vi "WriteFault.vi"(1 "Fault":T1 {"Severity" max=10}, 2 "FaultDevRef":T3) -> ()   [LabVIEW 2016]
uses:
  Fault_Fifos.ctl
  Faults.ctl
  Fault_Cluster.ctl
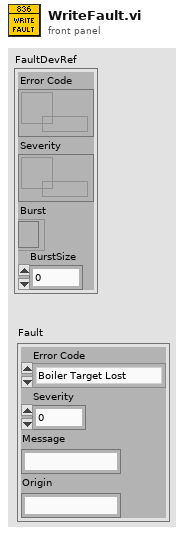
[diagram p1: front panel]
types:
  T1 = typedef "Fault_Cluster.ctl" = cluster{"Error Code":T2, "Severity":u32, "Message":string, "Origin":string}
  T2 = typedef "Faults.ctl" = enum16{"Boiler Target Lost", "Gerar Target Lost", "Body IMU Fault", "Turret IMU Fault"}
  T3 = typedef "Fault_Fifos.ctl" = cluster{"Error Code":refnum<k33>, "Severity":refnum<k33>, "Burst":refnum<k4>, "BurstSize":u32}
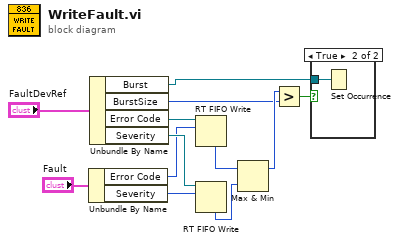
[diagram p0: block diagram]
diagram:
  n1 = Unbundle By Name("Fault") -> ("Error Code"=w8:T2, "Severity"=w7:u32)
  n2 = Unbundle By Name("FaultDevRef") -> ("Burst"=w1:refnum<k4>, "BurstSize"=w2:u32, "Error Code"=w11:refnum<k33>, "Severity"=w10:refnum<k33>)
  n3 = RT FIFO Write(0:w11, 1:w8) -> (7:w6:u32)  [unwired: 3 in, 3 out]
  n4 = RT FIFO Write(0:w10, 1:w7) -> (7:w5:u32)  [unwired: 3 in, 3 out]
  n5 = Max & Min(x=w6, y=w5) -> (max(x,y)=w4:u32)  [unwired: 1 out]
  n6 = Greater?(x=w4, y=w2) -> (0:w3:bool)
  n7 = case shown="True" w3 {
    tunnel: w1 -> [_ w13]
    frame False {
    }
    frame True {
      n8 = Set Occurrence(w13) -> ()
    }
  }
